vi "Flatten Value.vi"(0 "Int In":refnum<class "Integer.lvclass">, 11 "Error In":errorcluster) -> (4 "Int Out":refnum<class "Integer.lvclass">, 8 "Value":string, 15 "Error Out":errorcluster)   [LabVIEW 2016, in "Integer.lvclass"]
uses:
  Integer.lvclass
  Integer.lvclass/Integer.ctl
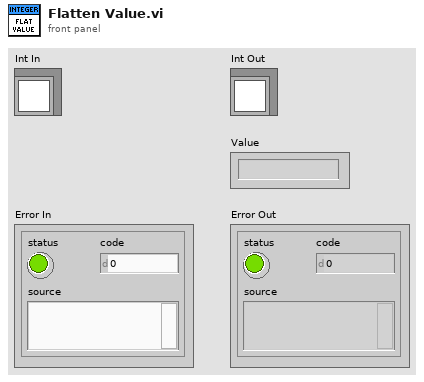
[diagram p1: front panel]
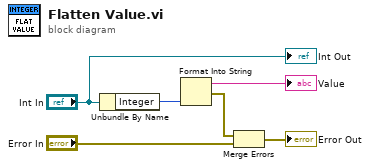
[diagram p0: block diagram]
diagram:
  n1 = Unbundle By Name("Int In") -> ("Integer"=w5:i64)
  n2 = Format Into String(w5) -> (resulting string=→"Value":string, error out=w3:errorcluster)  [unwired: 3 in]
  n3 = Merge Errors(w3, "Error In") -> (→"Error Out":errorcluster)
  "Int Out" <- "Int In"
